vi "Read Mod Freq.vi"(8 "error in (no error)":errorcluster, 11 "PAS Cell in":refnum<class "PAS Cell.lvclass">) -> (0 "error out":errorcluster, 2 "Mod Freq":sgl, 3 "PAS Cell out":refnum<class "PAS Cell.lvclass">)   [LabVIEW 2016, in "PAS Library.lvlib" / "PAS Cell.lvclass"]
uses:
  PAS Cell.lvclass
  PAS Cell.lvclass/PAS Cell.ctl
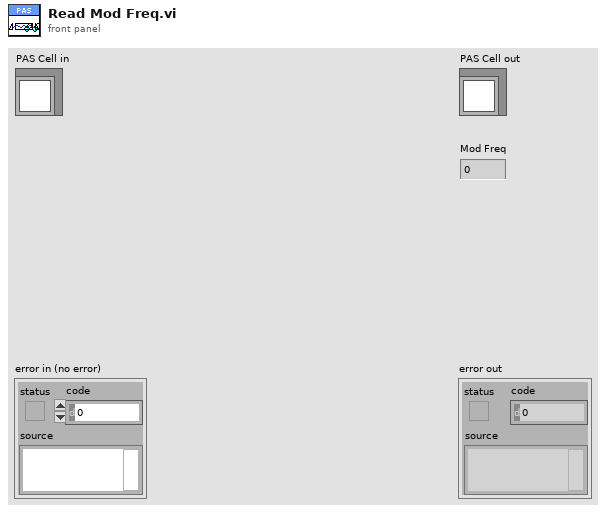
[diagram p1: front panel]
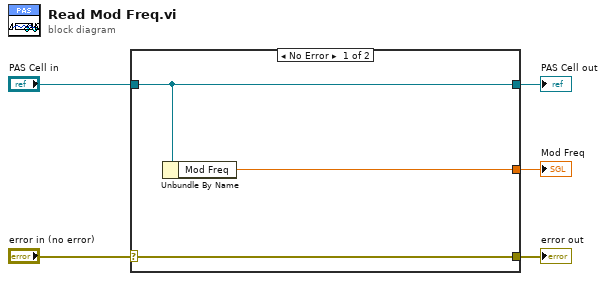
[diagram p0: block diagram]
diagram:
  n1 = case shown="No Error" "error in (no error)" {
    selector: "error in (no error)" -> [w8 w9]
    tunnel: [w8 w9] -> w4
    tunnel: [w7 w10] -> w2
    tunnel: "PAS Cell in" -> [w7 w10]
    tunnel: [w6 _] -> w1
    frame No Error {
      n2 = Unbundle By Name(w7) -> ("Mod Freq"=w6:sgl)
    }
    frame Error {
    }
  }
  "error out" <- w4
  "PAS Cell out" <- w2
  "Mod Freq" <- w1
